vi "WriteData.vi"(3 "Data In":T1) -> ()   [LabVIEW 2020]
uses:
  Ctrls/DataCluster.ctl
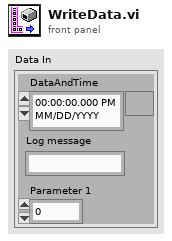
[diagram p1: front panel]
types:
  T1 = typedef "DataCluster.ctl" = cluster{"DataAndTime":timestamp, "Log message ":string, "Parameter 1":dbl}
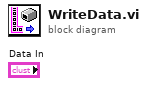
[diagram p0: block diagram]
diagram:
